vi "Shut Down.vi"(8 "error in (no error)":errorcluster, 11 "CCDCamera in":refnum<class "CCDCamera.lvclass">) -> (0 "error out":errorcluster, 3 "CCDCamera out":refnum<class "CCDCamera.lvclass">)   [LabVIEW 2018, in "CCDCamera.lvclass"]
doc: "This VI close the shutter, and then shutdown the camera."
uses:
  CCDCamera.lvclass
  CCDCamera.lvclass/CCDCamera.ctl
  <userlib>/atmcd32d.llb/Shutter_type typedef.ctl
  <userlib>/atmcd32d.llb/Shutter_mode typedef.ctl
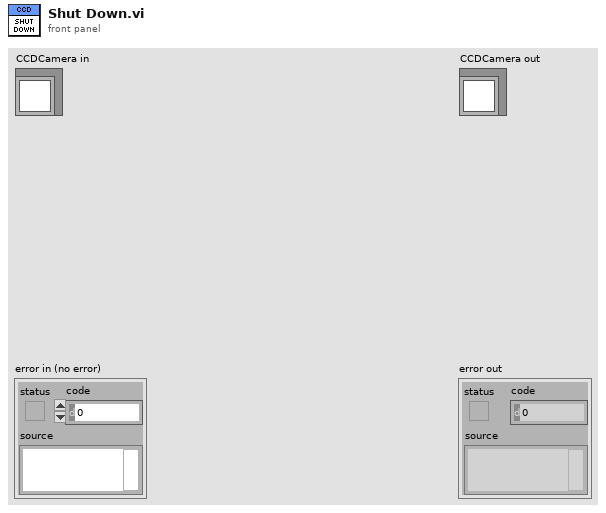
[diagram p1: front panel]
types:
  T1 = typedef "Shutter_mode typedef.ctl" = enum16{"Auto", "Open", "Close", "N/A (3)", "Open FVB Series", "Open Any Series"}
  T2 = typedef "Shutter_type typedef.ctl" = enum16{"TTL Low", "TTL High"}
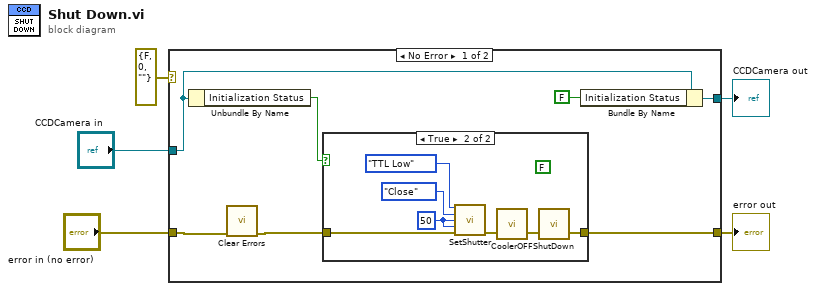
[diagram p0: block diagram]
diagram:
  n1 = case shown="No Error" errorcluster {"status"=FALSE, "code"=0, "source"=""} ("error IO") {
    selector: errorcluster {"status"=FALSE, "code"=0, "source"=""} ("error IO") -> [_ w22]
    tunnel: [w11 w22] -> w5
    tunnel: [w10 w21] -> w3
    tunnel: "CCDCamera in" -> [w8 w21]
    tunnel: "error in (no error)" -> [w7 _]
    frame No Error {
      n2 = Unbundle By Name(w8) -> ("Initialization Status"=w12:bool)
      n3 = call <vilib>:"Clear Errors.vi"("error in (no error)"=w7) -> ("error out"=w6:errorcluster)  [unwired: 5 in, 1 out]
      n4 = case shown="True" w12 {
        tunnel: [w13 w18] -> w11
        tunnel: w6 -> [w13 w17]
        frame False {
        }
        frame True {
          (unwired) FALSE ("Initialization Status")
          w14 = 50 ("closingtime")
          n5 = call <userlib>:"SetShutter.vi"("type"=Shutter_type_typedef."TTL Low", "mode"=Shutter_mode_typedef."Close", "closingtime"=w14, "openingtime"=w14, "error in (no error)"=w17) -> ("error out"=w20:errorcluster)  [unwired: 9 in, 1 out]
          n6 = call <userlib>:"CoolerOFF.vi"("error in (no error)"=w20) -> ("error out"=w19:errorcluster)  [unwired: 1 in, 1 out]
          n7 = call <userlib>:"ShutDown.vi"("error in (no error)"=w19) -> ("error out"=w18:errorcluster)  [unwired: 1 in, 1 out]
        }
      }
      n8 = Bundle By Name(cluster=w8, "Initialization Status"=FALSE) -> (w10:refnum<class "CCDCamera.lvclass">)
    }
    frame Error {
    }
  }
  "error out" <- w5
  "CCDCamera out" <- w3
